vi "verify parameter in range.vi"(8 "error in (no error)":errorcluster, 11 "Channel in":refnum<class "Channel.lvclass">) -> (0 "error out":errorcluster, 3 "Channel out":refnum<class "Channel.lvclass">)   [LabVIEW 2018, in "Channel.lvclass"]
uses:
  Channel.lvclass
  <vilib>/ErrorRing/Error Ring.xnode
  Sim_CCD/Sim_CCD.lvclass
panel:
  in  "parameter name":string
  in  "upper limit":dbl format="%#_13g"
  in  "value":dbl format="%#_13g"
  in  "lower limit":dbl format="%#_13g"
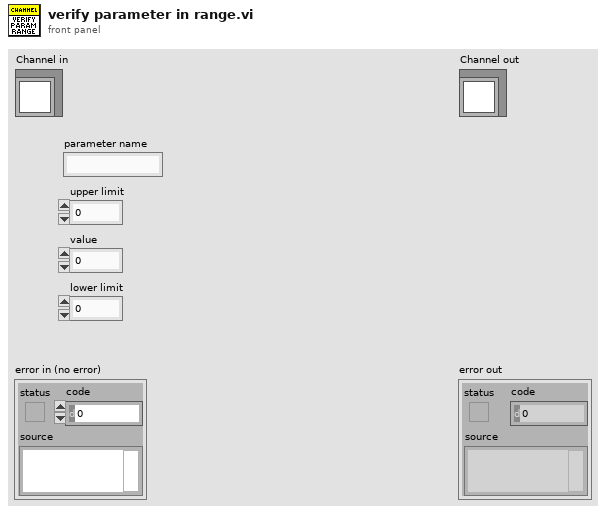
[diagram p1: front panel]
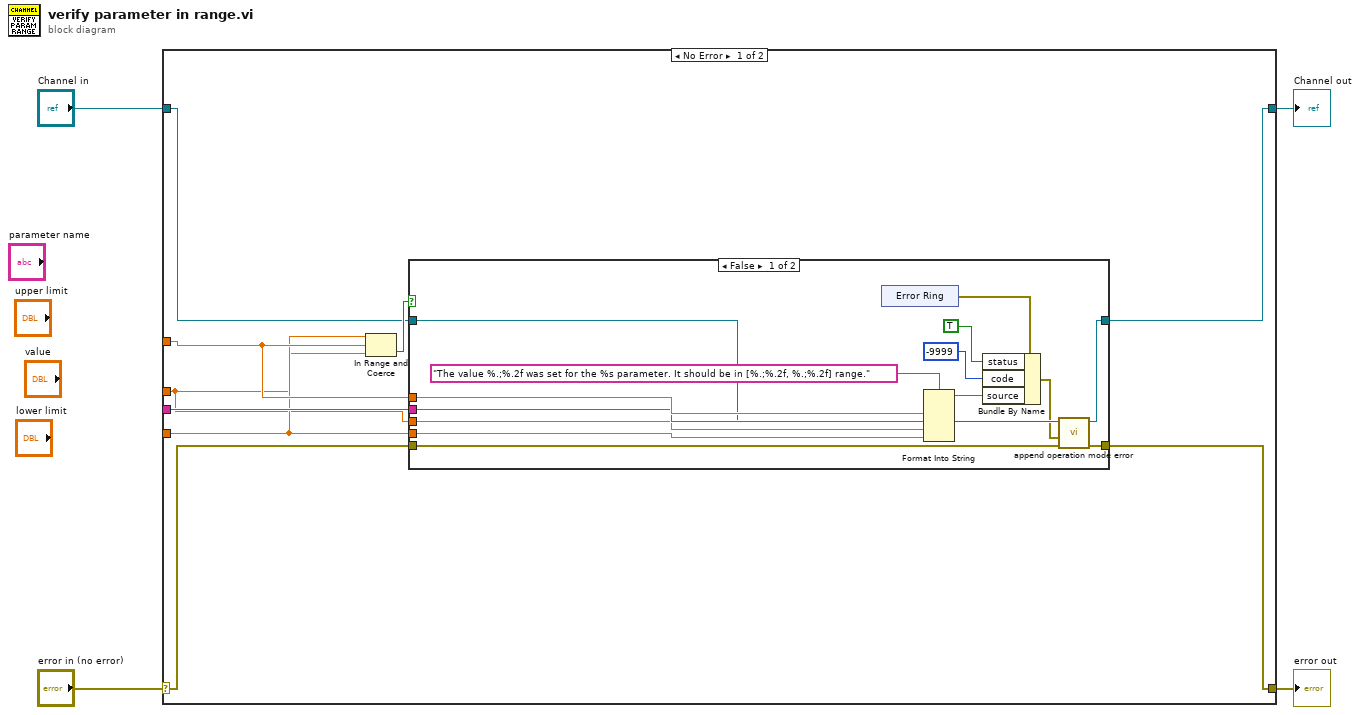
[diagram p0: block diagram]
diagram:
  n1 = case shown="No Error" "error in (no error)" {
    selector: "error in (no error)" -> [w16 w36]
    tunnel: [w15 w36] -> w7
    tunnel: [w13 w35] -> w5
    tunnel: "Channel in" -> [w14 w35]
    tunnel: [w12 _] -> w4
    tunnel: [w11 _] -> w3
    tunnel: [w10 _] -> w2
    tunnel: [w9 _] -> w1
    frame No Error {
      n2 = In Range and Coerce(upper limit=w10, x=w11, lower limit=w9) -> (In Range?=w17:bool)  [unwired: 1 out]
      n3 = case shown="False" w17 {
        tunnel: [w22 w34] -> w13
        tunnel: w14 -> [w21 w34]
        tunnel: w12 -> [w25 _]
        tunnel: w16 -> [w20 w33]
        tunnel: [w19 w33] -> w15
        tunnel: w11 -> [w27 _]
        tunnel: w9 -> [w24 _]
        tunnel: w10 -> [w23 _]
        frame False {
          n4 = xnode "Error Ring"() -> ("error out"=w31:errorcluster)
          n5 = Format Into String(format string="The value %.;%.2f was set for the %s parameter. It should be in [%.;%.2f, %.;%.2f] range." ("string"), w27, w25, w24, w23) -> (resulting string=w26:string)  [unwired: 2 in, 1 out]
          n6 = Bundle By Name(cluster=w31, "status"=TRUE, "code"=-9999, "source"=w26) -> (w18:errorcluster)
          n7 = call "append operation mode error.vi"("error in (no error)"=w20, 9:w18, "Simulated_CCD_Camera in"=w21) -> ("error out"=w19:errorcluster, "Simulated_CCD_Camera out"=w22:refnum<class "Sim_CCD.lvclass">)  [unwired: 7 in]
        }
        frame True {
        }
      }
    }
    frame Error {
    }
  }
  "error out" <- w7
  "Channel out" <- w5
